vi "VI Documentation Tool.vi"   [LabVIEW 2013]
uses:
  VI properties editor/Update VI Properties.vi
  VI properties editor/update vi properties.lvlib
types:
  T1 = enum32{"Invalid", "Standard", "Closed", "Hidden", "Minimized", "Maximized"}
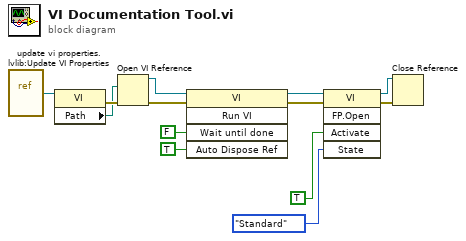
[diagram p0: block diagram]
diagram:
  n1 = vi-ref "update vi properties.lvlib:Update VI Properties.vi"() -> (w13:refnum<vi>)
  n2 = property class="VI"(reference=w13) -> (error out=w12:errorcluster, "Path"=w11:path)  [unwired: 1 in, 1 out]
  n3 = Open VI Reference(vi path=w11, error in (no error)=w12) -> (vi reference=w7:refnum<vi>, error out=w10:errorcluster)  [unwired: 4 in]
  n4 = invoke class="VI" method="Run VI"(reference=w7, error in=w10, "Wait until done"=FALSE ("Wait Until Done"), "Auto Dispose Ref"=TRUE ("Auto Dispose Reference")) -> (reference out=w6:refnum<vi>, error out=w8:errorcluster)  [unwired: 1 in, 3 out]
  n5 = invoke class="VI" method="FP.Open"(reference=w6, error in=w8, "Activate"=TRUE ("Activate?"), "State"=T1."Standard") -> (reference out=w1:refnum<vi>, error out=w2:errorcluster)  [unwired: 1 in, 3 out]
  n6 = Close Reference(reference=w1, error in (no error)=w2) -> ()  [unwired: 1 out]
